vi "Handle Message.vi"(8 "error in":errorcluster, 11 "Serial FPGA in":refnum<class "Serial FPGA.lvclass">) -> (0 "error out":errorcluster, 3 "Serial FPGA out":refnum<class "Serial FPGA.lvclass">)   [LabVIEW 2013, in "Serial FPGA.lvclass"]
uses:
  Serial FPGA.lvclass
  Message/Serial Message.lvclass
  Serial FPGA.lvclass/Serial FPGA.ctl
  <vilib>/rvi/eio/common/nirviEmuTemplateMethod_errors.vi
  <vilib>/eio/EIOMethodNode/EIOMethodNode.xnode
panel:
  in  "MSG In":refnum<class "Serial Message.lvclass">
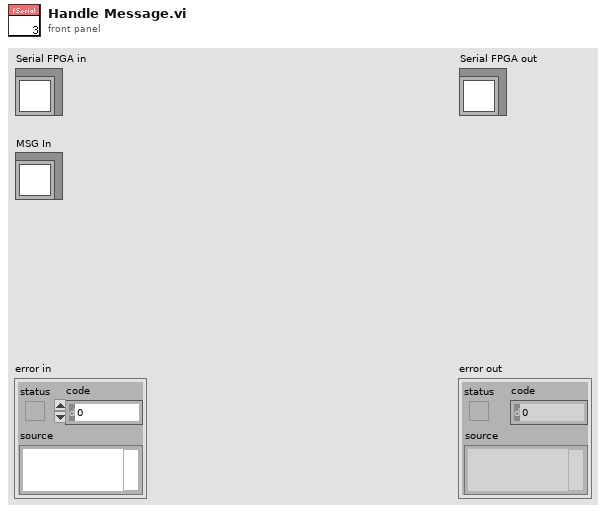
[diagram p1: front panel]
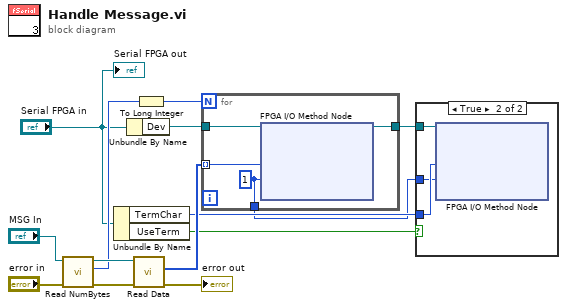
[diagram p0: block diagram]
diagram:
  n1 = call "Read NumBytes.vi"("error in (no error)"="error in", "Serial Message in"="MSG In") -> ("error out"=w7:errorcluster, "NumBytes"=w8:u8, "Serial Message out"=w11:refnum<class "Serial Message.lvclass">)  [unwired: 7 in]
  n2 = Unbundle By Name("Serial FPGA in") -> ("TermChar"=w3:i16, "UseTerm"=w2:bool)
  n3 = Unbundle By Name("Serial FPGA in") -> ("Dev"=w6:refnum<k21>)
  n4 = call "Read Data.vi"("error in (no error)"=w7, "Serial Message in"=w11) -> ("error out"=→"error out":errorcluster, "Data"=w10:u8[])  [unwired: 7 in, 1 out]
  n5 = To Long Integer(number=w8) -> (32bit integer=w9:i32)
  n6 = for {
    N: w9 -> [_]
    tunnel: w10 -> [w17] mode=indexing
    tunnel: [w15] -> w1
    tunnel: w6 -> [w18]
    tunnel: [w16] -> w5
    w15 = 1 ("Timeout (ms)")
    n7 = xnode "FPGA I/O Method Node"("FPGA I/O In"=w18, "Data"=w17, "Timeout (ms)"=w15) -> ("FPGA I/O Out"=w16:refnum<k21>)  [unwired: 1 out]
  }
  n8 = case shown="True" w2 {
    tunnel: w5 -> [_ w21]
    tunnel: w3 -> [_ w20]
    tunnel: w1 -> [_ w19]
    frame False {
    }
    frame True {
      n9 = xnode "FPGA I/O Method Node"("FPGA I/O In"=w21, "Data"=w20, "Timeout (ms)"=w19) -> ()  [unwired: 2 out]
    }
  }
  "Serial FPGA out" <- "Serial FPGA in"
